vi "AIO Synchronize.vi"(2 "rate":dbl=25600.0, 3 "number of samples":i32=260000, 4 "timeout (s)":dbl=15.0 format="%0.2f", 5 "error in":errorcluster, 7 "stop (T)":bool=TRUE, 10 "device name":tag="Dev1") -> (14 "task out":refnum<k21>, 15 "data":dynamicdata(graph), 19 "error out":errorcluster)   [LabVIEW 2013]
doc: "Creates, edits, and runs tasks using NI-DAQmx. Refer to the NI-DAQmx Readme for a complete listing of devices NI-DAQmx supports.\n\nWhen you place this Express VI on the block diagram, the DAQ Assistant launches to create a new task. After you create a task, you can double-click the DAQ Assistant Express VI to edit that task. For continuous measurement or generation, place a while loop around the DAQ Assistant Express VI.\n\nFor continuous single-point input or output, the DAQ Assistant Express VI might not provide optimal performance. Refer to the Cont Acq&Graph Voltage-Single Point Optimization VI in examples\\DAQmx\\Analog In\\Measure Voltage.llb for an example of techniques to create higher-performance, single-point I/O applications."
uses:
  <vilib>/DAQmx/read.llb/DAQmx Read.vi
  <vilib>/DAQmx/read.llb/DAQmx Read (Analog 1D Wfm NChan NSamp).vi
  <vilib>/DAQmx/create/channels.llb/DAQmx Create Channel (TEDS-AI-Acceleration-Accelerometer).vi
  <vilib>/DAQmx/create/channels.llb/DAQmx Create Channel (AI-Acceleration-Accelerometer).vi
  <vilib>/DAQmx/configure/timing.llb/DAQmx Timing (Sample Clock).vi
  <vilib>/DAQmx/configure/trigger.llb/DAQmx Start Trigger (Digital Edge).vi
  <vilib>/DAQmx/miscellaneous.llb/DAQmx Fill In Error Info.vi
  <resource>/objmgr/daqmx.rc
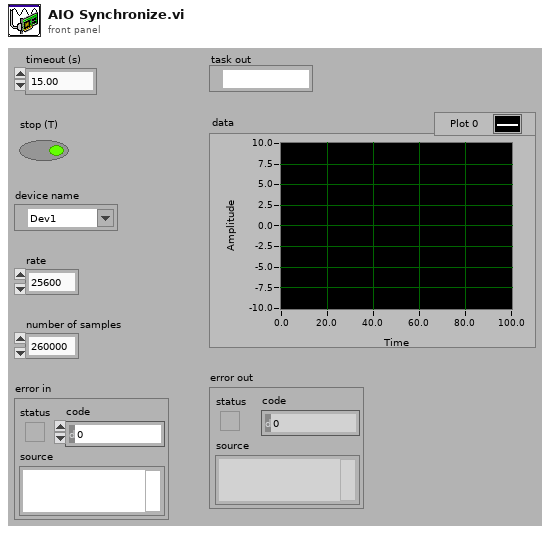
[diagram p1: front panel]
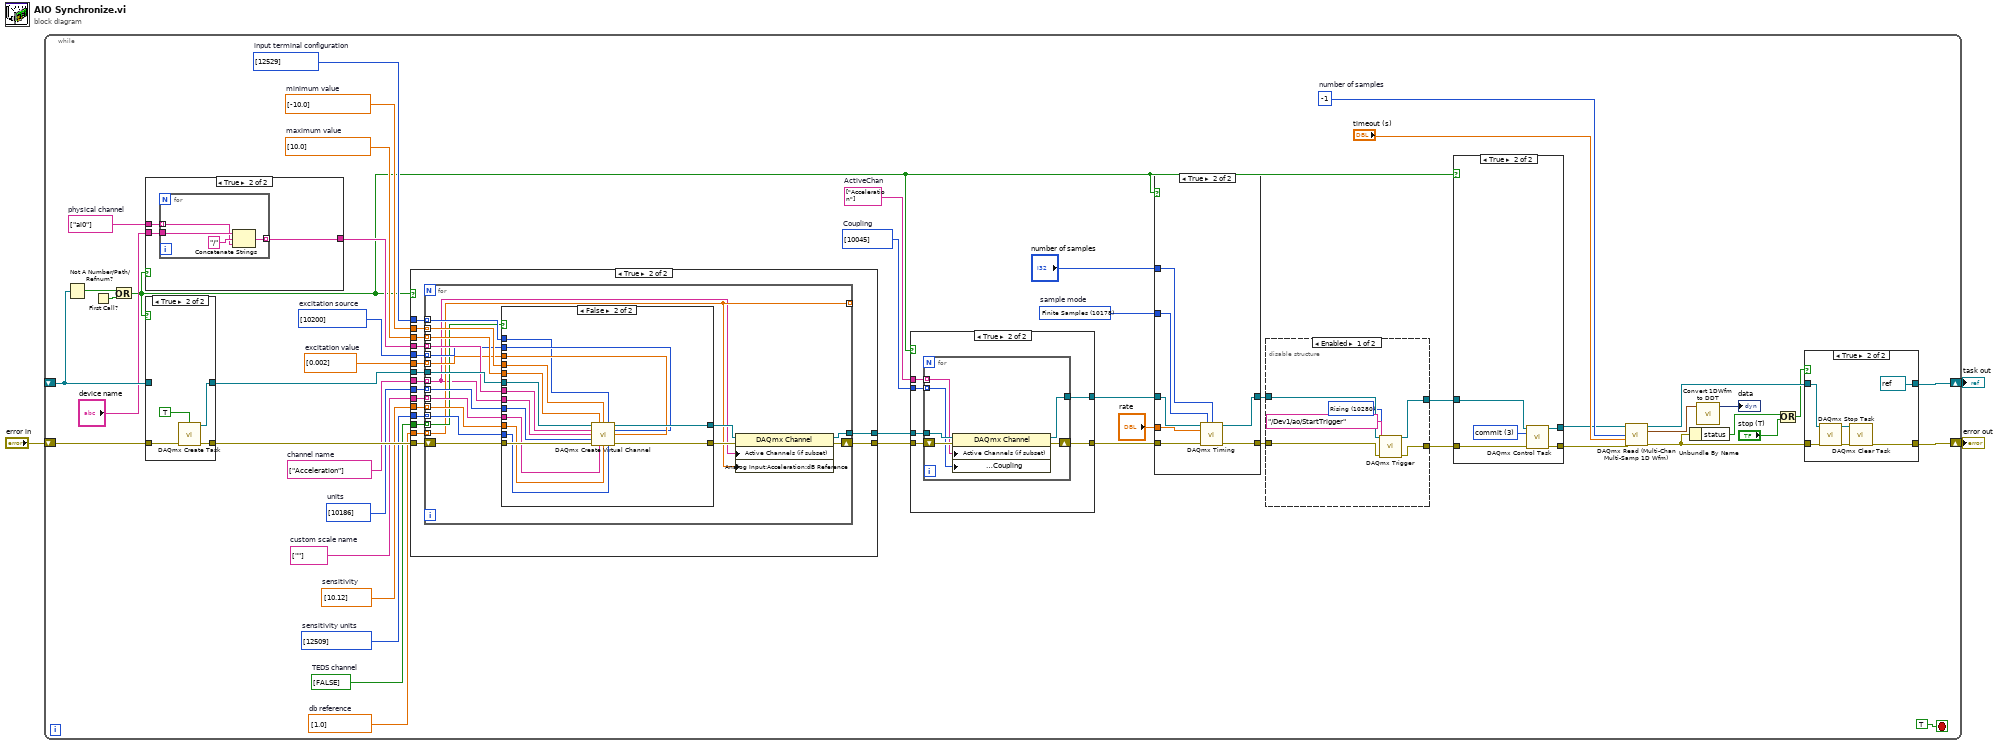
[diagram p0: block diagram]
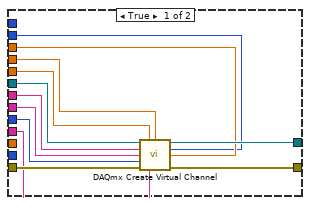
[diagram p8: hidden frame]
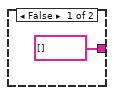
[diagram p9: hidden frame]
diagram:
  n1 = while {
    shift-right: [w16] -> w1
    shift-left: _ -> [w49]
    shift-right: [w14] -> w2
    shift-left: "error in" -> [w50]
    stop <- TRUE stop-if-true
    w20 = -1  # number of samples
    w22 = 10178 items=["Finite Samples"=10178, "Continuous Samples"=10123, "Hardware Timed Single Point"=12522]  # sample mode
    w30 = string[] ["Acceleration"]  # ActiveChan
    w29 = i32[] [10045] items=["AC"=10045, "DC"=10050, "GND"=10066]  # Coupling
    w31 = dbl[] [1.0]  # db reference
    w32 = bool[] [FALSE]  # TEDS channel
    w33 = i32[] [12529] items=["default"=-1, "RSE"=10083, "NRSE"=10078, "Differential"=10106, "Pseudodifferential"=12529]  # input terminal configuration
    w35 = dbl[] [10.12]  # sensitivity
    w36 = i32[] [10200] items=["Internal"=10200, "External"=10167, "None"=10230]  # excitation source
    w34 = i32[] [12509] items=["mVolts/g"=12509, "Volts/g"=12510]  # sensitivity units
    w37 = dbl[] [0.002]  # excitation value
    w38 = string[] [""]  # custom scale name
    w39 = i32[] [10186] items=["g"=10186, "m/s^2"=12470, "From Custom Scale"=10065]  # units
    w40 = string[] ["Acceleration"]  # channel name
    w42 = dbl[] [10.0]  # maximum value
    w43 = dbl[] [-10.0]  # minimum value
    w46 = string[] ["ai0"]  # physical channel
    n2 = Not A Number/Path/Refnum?(number/path/refnum=w49) -> (NaN/Path/Refnum?=w48:bool)
    n3 = First Call?() -> (First Call?: T/F=w51:bool)
    n4 = Or(x=w48, y=w51) -> (x .or. y?=w21:bool)
    n5 = case shown="True" w21 {
      tunnel: [string[] [] w167] -> w41
      tunnel: "device name" -> [_ w166]
      tunnel: w46 -> [_ w165]
      frame False {
      }
      frame True {
        n6 = for {
          tunnel: [w171] -> w167 mode=indexing
          tunnel: w166 -> [w170]
          tunnel: w165 -> [w168] mode=indexing
          n7 = Concatenate Strings(w170, "/" ("string"), w168) -> (w171:string)
        }
      }
    }
    n8 = case shown="True" w21 {
      tunnel: [w173 w177] -> w45
      tunnel: w49 -> [w173 _]
      tunnel: [w172 w176] -> w44
      tunnel: w50 -> [w172 w174]
      frame False {
      }
      frame True {
        n9 = call <vilib>:"DAQmx Create Task.vi"("auto cleanup"=TRUE, "error in"=w174) -> ("task out"=w177:refnum<k21>, "error out"=w176:errorcluster)  [unwired: 12 in]
      }
    }
    n10 = case shown="True" w21 {
      tunnel: [w100 w115] -> w28
      tunnel: w45 -> [w100 w117]
      tunnel: [w99 w114] -> w27
      tunnel: w44 -> [w99 w116]
      tunnel: w43 -> [_ w113]
      tunnel: w42 -> [_ w112]
      tunnel: w41 -> [_ w111]
      tunnel: w40 -> [_ w110]
      tunnel: w39 -> [_ w109]
      tunnel: w38 -> [_ w108]
      tunnel: w37 -> [_ w107]
      tunnel: w36 -> [_ w106]
      tunnel: w35 -> [_ w105]
      tunnel: w34 -> [_ w104]
      tunnel: w33 -> [_ w103]
      tunnel: w32 -> [_ w102]
      tunnel: w31 -> [_ w101]
      frame False {
      }
      frame True {
        n11 = for {
          tunnel: w117 -> [w136]
          tunnel: [w122] -> w115
          tunnel: w113 -> [w134] mode=indexing
          tunnel: w112 -> [w133] mode=indexing
          tunnel: w111 -> [w132] mode=indexing
          tunnel: w110 -> [w118] mode=indexing
          tunnel: w109 -> [w131] mode=indexing
          tunnel: w108 -> [w130] mode=indexing
          shift-right: [w121] -> w114
          shift-left: w116 -> [w135]
          tunnel: w107 -> [w129] mode=indexing
          tunnel: w106 -> [w128] mode=indexing
          tunnel: w105 -> [w127] mode=indexing
          tunnel: w104 -> [w126] mode=indexing
          tunnel: w103 -> [w125] mode=indexing
          tunnel: w102 -> [w124] mode=indexing
          tunnel: [w119] -> _ mode=indexing
          tunnel: w101 -> [w119] mode=indexing
          n12 = case shown="False" w124 {
            tunnel: w136 -> [w148 w163]
            tunnel: w135 -> [w147 w162]
            tunnel: [w146 w161] -> w123
            tunnel: [w145 w160] -> w120
            tunnel: w134 -> [w144 w159]
            tunnel: w133 -> [w143 w158]
            tunnel: w132 -> [w142 w157]
            tunnel: w118 -> [w141 w156]
            tunnel: w131 -> [w140 w155]
            tunnel: w130 -> [w139 w154]
            tunnel: w129 -> [w138 w153]
            tunnel: w128 -> [w137 w152]
            tunnel: w127 -> [_ w151]
            tunnel: w126 -> [_ w150]
            tunnel: w125 -> [_ w149]
            frame True {
              n13 = call-poly <vilib>:"DAQmx Create Virtual Channel.vi"("task in"=w148, "maximum value"=w143, "minimum value"=w144, "physical channels"=w142, "current excitation source"=w137, "name to assign"=w141, "current excitation value"=w138, "units"=w140, "error in"=w147, "custom scale name"=w139) -> ("task out"=w146:refnum<k21>, "error out"=w145:errorcluster)  [unwired: 4 in]
            }
            frame False {
              n14 = call-poly <vilib>:"DAQmx Create Virtual Channel.vi"("task in"=w163, "maximum value"=w158, "minimum value"=w159, "input terminal configuration"=w149, "physical channels"=w157, "current excitation source"=w152, "name to assign"=w156, "current excitation value"=w153, "units"=w155, "error in"=w162, "custom scale name"=w154, "sensitivity"=w151, "sensitivity units"=w150) -> ("task out"=w161:refnum<k21>, "error out"=w160:errorcluster)  [unwired: 1 in]
            }
          }
          n15 = property class="DAQmx Channel"(reference=w123, error in=w120, "Active Channels (if subset)"=w118, "Analog Input:Acceleration:dB Reference"=w119) -> (reference out=w122:refnum<k21>, error out=w121:errorcluster)
        }
      }
    }
    n16 = case shown="True" w21 {
      tunnel: w28 -> [w86 w92]
      tunnel: w27 -> [w85 w91]
      tunnel: [w86 w90] -> w26
      tunnel: [w85 w89] -> w25
      tunnel: w30 -> [_ w88]
      tunnel: w29 -> [_ w87]
      frame False {
      }
      frame True {
        n17 = for {
          tunnel: w92 -> [w98]
          tunnel: [w96] -> w90
          tunnel: w88 -> [w94] mode=indexing
          shift-right: [w95] -> w89
          shift-left: w91 -> [w97]
          tunnel: w87 -> [w93] mode=indexing
          n18 = property class="DAQmx Channel"(reference=w98, error in=w97, "Active Channels (if subset)"=w94, "Analog Input:General Properties:Input Configuration:Coupling"=w93) -> (reference out=w96:refnum<k21>, error out=w95:errorcluster)
        }
      }
    }
    n19 = case shown="True" w21 {
      tunnel: [w77 w79] -> w7
      tunnel: w26 -> [w77 w82]
      tunnel: [w76 w78] -> w6
      tunnel: w25 -> [w76 w80]
      tunnel: "number of samples" -> [_ w84]
      tunnel: w22 -> [_ w83]
      tunnel: "rate" -> [_ w81]
      frame False {
      }
      frame True {
        n20 = call-poly <vilib>:"DAQmx Timing.vi"("task/channels in"=w82, "sample mode"=w83, "samples per channel"=w84, "rate"=w81, "error in"=w80) -> ("task out"=w79:refnum<k21>, "error out"=w78:errorcluster)  [unwired: 9 in]
      }
    }
    n21 = disable-structure shown="Enabled" {
      disable-tunnel: w7 -> [w57 w60]
      disable-tunnel: w6 -> [w56 w59]
      disable-tunnel: [w55 w59] -> w5
      disable-tunnel: [w54 w60] -> w4
      frame Enabled {
        w53 = 10280 items=["Rising"=10280, "Falling"=10171] ("edge")
        n22 = call-poly <vilib>:"DAQmx Trigger.vi"("task/channels in"=w57, "source"=tag "/Dev1/ao/StartTrigger", "edge"=w53, "error in"=w56) -> ("task out"=w54:refnum<k21>, "error out"=w55:errorcluster)  [unwired: 10 in]
      }
      frame Disabled {
      }
    }
    n23 = case shown="True" w21 {
      tunnel: [w70 w74] -> w9
      tunnel: w4 -> [w70 w75]
      tunnel: [w69 w72] -> w8
      tunnel: w5 -> [w69 w73]
      frame False {
      }
      frame True {
        w71 = 3 items=["verify"=2, "reserve"=4, "commit"=3, "unreserve"=5, "abort"=6] ("action")
        n24 = call <vilib>:"DAQmx Control Task.vi"("task/channels in"=w75, "action"=w71, "error in"=w73) -> ("task out"=w74:refnum<k21>, "error out"=w72:errorcluster)  [unwired: 11 in]
      }
    }
    n25 = call-poly "DAQmx Read (Multi-Chan Multi-Samp 1D Wfm).vi"("task/channels in"=w9, "number of samples per channel"=w20, "timeout"="timeout (s)", "error in"=w8) -> ("task out"=w15:refnum<k21>, "data"=w19:waveform(dbl)[], "error out"=w13:errorcluster)  [unwired: 9 in]
    n26 = Unbundle By Name(w13) -> ("status"=w12:bool)
    n27 = call <vilib>:"Convert 1DWfm to DDT.vi"("Array of Waveforms"=w19) -> ("Dynamic Data Type"=→"data":dynamicdata)  [unwired: 3 in]
    n28 = Or(x=w12, y="stop (T)") -> (x .or. y?=w10:bool)
    n29 = case shown="True" w10 {
      tunnel: [w62 refnum<k21> refnum ("task in")] -> w16
      tunnel: w15 -> [w62 w68]
      tunnel: [w61 w65] -> w14
      tunnel: w13 -> [w61 w67]
      frame False {
      }
      frame True {
        n30 = call <vilib>:"DAQmx Stop Task.vi"("task/channels in"=w68, "error in"=w67) -> ("task out"=w64:refnum<k21>, "error out"=w66:errorcluster)  [unwired: 12 in]
        n31 = call <vilib>:"DAQmx Clear Task.vi"("task in"=w64, "error in"=w66) -> ("error out"=w65:errorcluster)  [unwired: 13 in]
      }
    }
  }
  "error out" <- w2
  "task out" <- w1
